vi "svfa_Peak Hold Array.vi"(6 "averages completed in":dbl, 7 "processing control":T1(ring), 8 "number of averages":u32, 10 "previous peak array":dbl[](array[numeric]) format="%.2f", 11 "array":dbl[](array[numeric]) format="%.2f") -> (1 "averaging done":bool, 2 "averages completed out":dbl, 3 "peak array":dbl[](array[numeric]) format="%.2f")   [LabVIEW 2017]
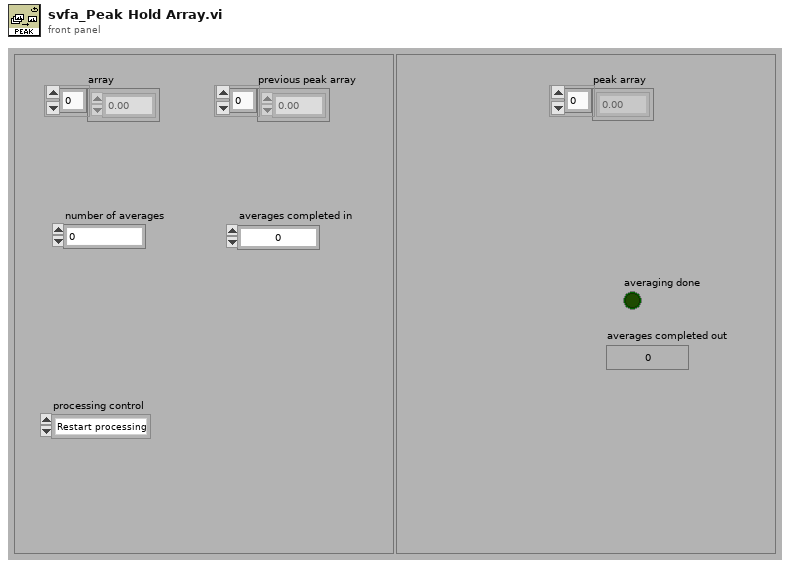
[diagram p1: front panel]
types:
  T1 = enum16{"Restart processing", "Continue processing", "Skip processing"}
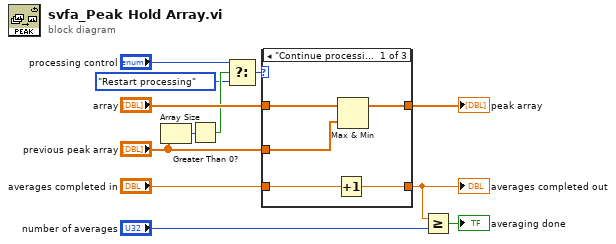
[diagram p0: block diagram]
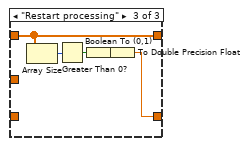
[diagram p3: hidden frame]
diagram:
  n1 = Array Size(array="previous peak array") -> (size(s)=w1:i32)
  n2 = Greater Than 0?(x=w1) -> (x > 0?=w6:bool)
  n3 = Select(t="processing control", s=w6, f=T1."Restart processing") -> (s? t:f=w3:T1)
  n4 = case shown="\"Continue processing\"" w3 {
    tunnel: [w17 w19 w20] -> w10
    tunnel: "averages completed in" -> [w16 w19 _]
    tunnel: [w15 w18 w23] -> w8
    tunnel: "array" -> [w14 _ w23]
    tunnel: "previous peak array" -> [w13 w18 _]
    frame "Continue processing" {
      n5 = Increment(x=w16) -> (x+1=w17:dbl)
      n6 = Max & Min(x=w14, y=w13) -> (max(x,y)=w15:dbl[])  [unwired: 1 out]
    }
    frame "Skip processing" {
    }
    frame "Restart processing" {
      n7 = Array Size(array=w23) -> (size(s)=w24:i32)
      n8 = Greater Than 0?(x=w24) -> (x > 0?=w22:bool)
      n9 = Boolean To (0,1)(Boolean=w22) -> (0, 1=w21:i16)
      n10 = To Double Precision Float(number=w21) -> (double precision float=w20:dbl)
    }
  }
  "averages completed out" <- w10
  "peak array" <- w8
  n11 = Greater Or Equal?(x=w10, y="number of averages") -> (x >= y?=→"averaging done":bool)
